vi "Collect file info metadata.vi"(0 "reference in":refnum<class "metadata.lvclass">, 5 "error in (no error)":errorcluster) -> (14 "reference out":refnum<class "metadata.lvclass">, 16 "Metadata":T1, 19 "error out":errorcluster)   [LabVIEW 2019, in "metadata.lvclass"]
uses:
  metadata.lvclass
  Metadata output --cluster.ctl
  Write time and date string --constant.ctl
panel:
  out "Property Names":string[](array[string])
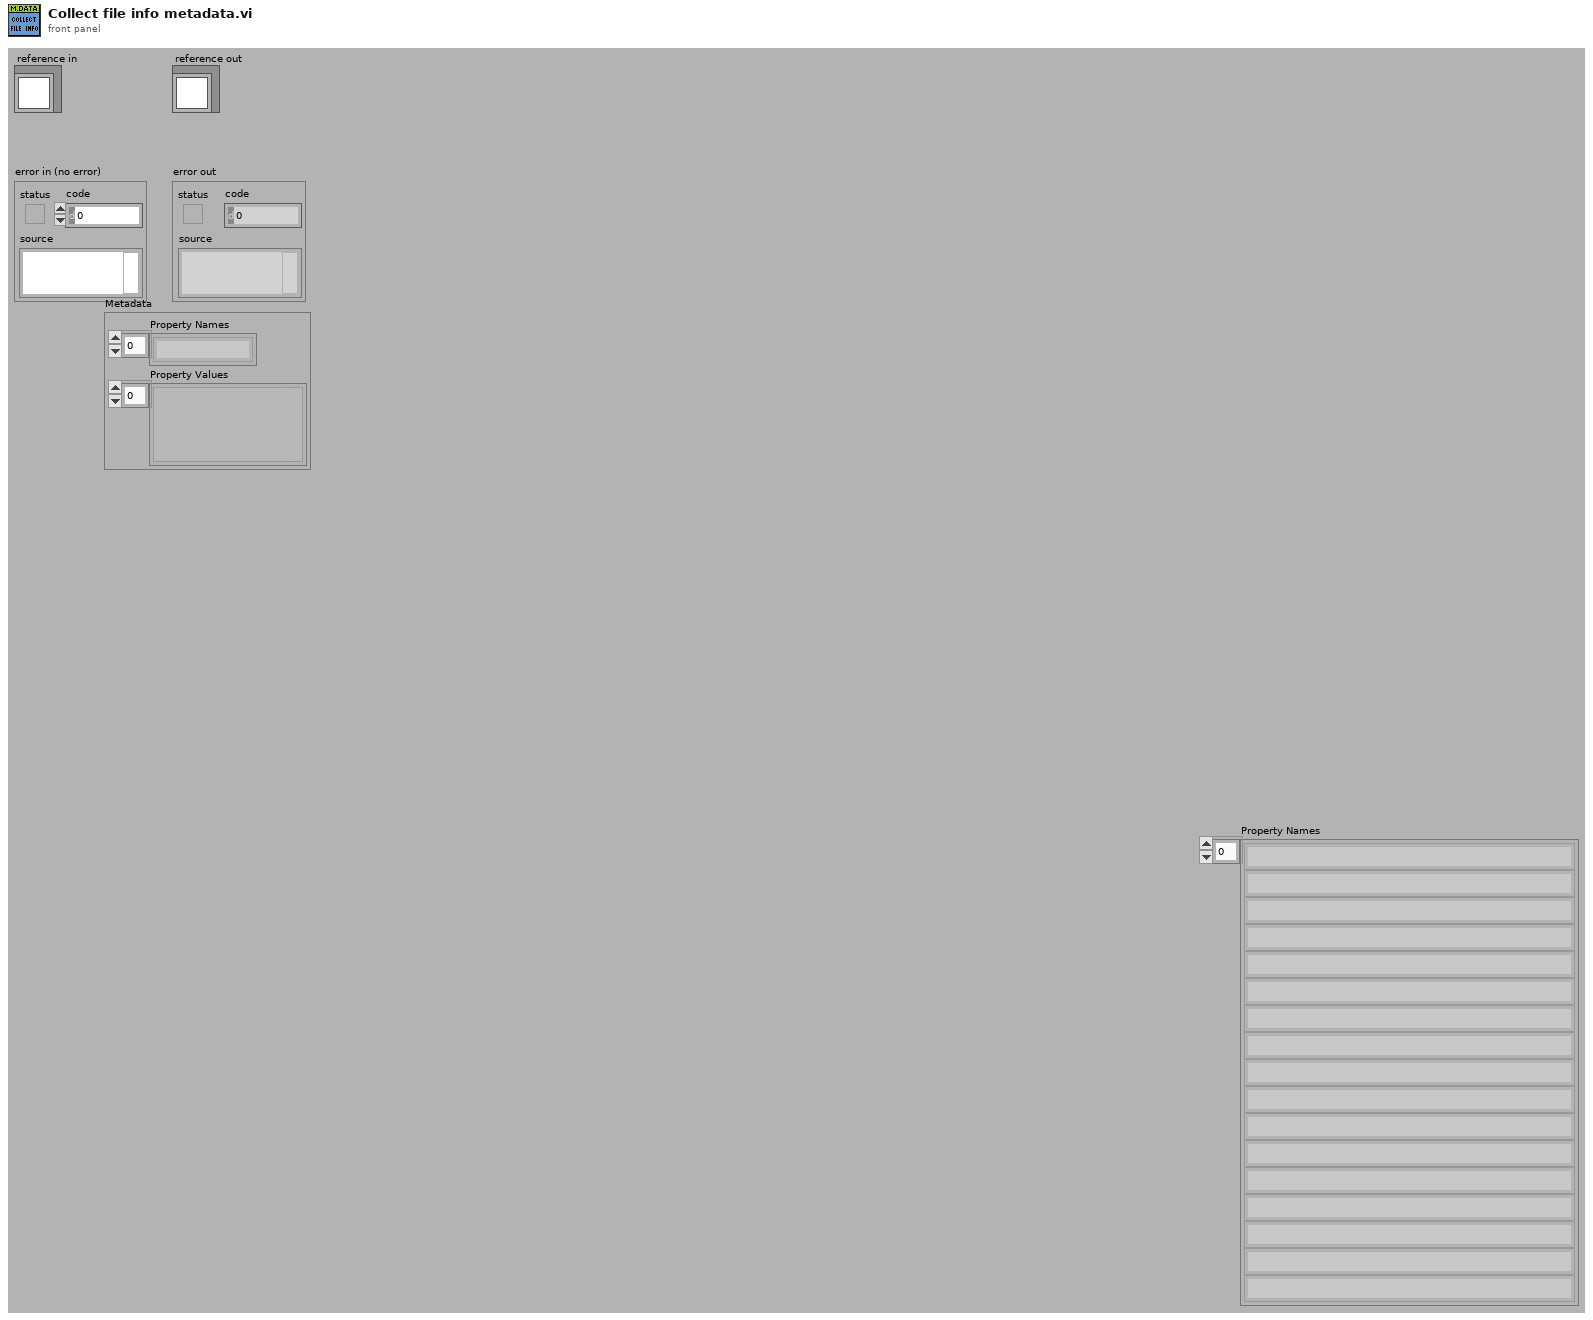
[diagram p1: front panel]
types:
  T1 = typedef "metadata.lvclass/Metadata output --cluster.ctl" = cluster{"Property Names":string[], "Property Values":variant[]}
  T2 = typedef "metadata.lvclass/Write time and date string --constant.ctl" = string
  T3 = typedef "metadata.lvclass/ObjectAttributes.ctl" = cluster{"MyAttribute":dbl, "System Control":T4, "file info":T5, "Sample info":T6, "Cantilever info":T7, "XYZ piezos":T8, "Mapping":T9, "Fcurve segment":T10[], "Fast fpga segment":T12, "Chirp":T13, "precision (6)":i16, "width (-)":i16, "Metadata":T1, "config filepath":path, "Section names []":string[], "Property names []":string[], "nb elements":u16}
  T4 = typedef "metadata.lvclass/System control parameters.ctl" = cluster{"FPGA SW version":string, "TDMS file version":string, "Instrument":string, "Instrument model":string, "Instrument scanner":string, "Instrument clockrate (Mhz)":string, "Instrument tick time (us)":string}
  T5 = typedef "metadata.lvclass/File info parameters.ctl" = cluster{"Time Stamp":timestamp, "Filename":string, "Filepath":path, "User":string, "Experiment_name":string, "Curve_id":string, "number_segments":u8, "number_consecutive_scans":u32}
  T6 = typedef "metadata.lvclass/Sample info parameters.ctl" = cluster{"Sample name":string, "Sample species":string}
  T7 = typedef "metadata.lvclass/Cantilever info parameters.ctl" = cluster{"spring constant calib method":string, "invOLS calib method":string, "thermal calib deflection channel":string, "model":string, "shape":string, "tip geometry":string, "Laser sum (V)":dbl, "Laser power (mA)":dbl, "invOLS_(nm/V)":dbl, "spring constant nominal (N/m)":dbl, "spring constant calib (N/m)":dbl, "resosnance frequency air calib (Hz)":dbl, "resosnance frequency calib (Hz)":dbl, "quality factor":dbl, "Acoefficident_GCI_(nN.s^1.3/m)":dbl, "half angle (deg)":dbl, "tip radius (m)":dbl, "tip height (m)":dbl, "system mount angle (deg)":dbl}
  T8 = typedef "metadata.lvclass/XYZ piezos parameters.ctl" = cluster{"X stage piezo sensitivity (nm/V)":dbl, "X stage piezo gain":dbl, "X velocity (V/tick)":dbl, "X closed loop":bool, "Y stage piezo sensitivity (nm/V)":dbl, "Y stage piezo gain":dbl, "Y velocity (V/tick)":dbl, "Y closed loop":bool, "Z stage piezo sensitivity (nm/V)":dbl, "Z stage piezo gain":dbl, "Z closed loop":bool, "X position (V)":dbl, "Y position (V)":dbl}
  T9 = typedef "metadata.lvclass/Mapping parameters.ctl" = cluster{"Mapping":bool, "index":u16, "position row":u16, "position column":u16, "next position row":i16, "next position column":i16, "X initial position (V)":dbl, "Y initial position (V)":dbl, "X step size (V)":dbl, "Y step size (V)":dbl}
  T10 = typedef "metadata.lvclass/Fcurve segment.ctl" = cluster{"type":T11, "fast_fpga_trigger":bool, "nb":u8, "duration (ticks)":i64, "nb points":i32, "sampling rate (S/s)":u32, "Zpiezo control out":string, "initial deflection (V)":dbl, "relative setpoint":bool, "setpoint on":bool, "setpoint (V)":dbl, "setpoint trigger channel":string, "velocity (V/tick)":dbl, "Z position setpoint trigger (V)":dbl, "Z retract length (V)":dbl, "dec factor":u32}
  T11 = typedef "metadata.lvclass/Segment type--combobox.ctl" = string
  T12 = typedef "metadata.lvclass/fast fpga segment parameters.ctl" = cluster{"Fast start time trigger":timestamp, "nb_points":u32, "sampling_rate_(S/s)":u32, "duration_(ticks)":u32}
  T13 = typedef "metadata.lvclass/Chirp added parameters.ctl" = cluster{"f start (Hz)":dbl, "f end (Hz)":dbl, "Sweep type":string}
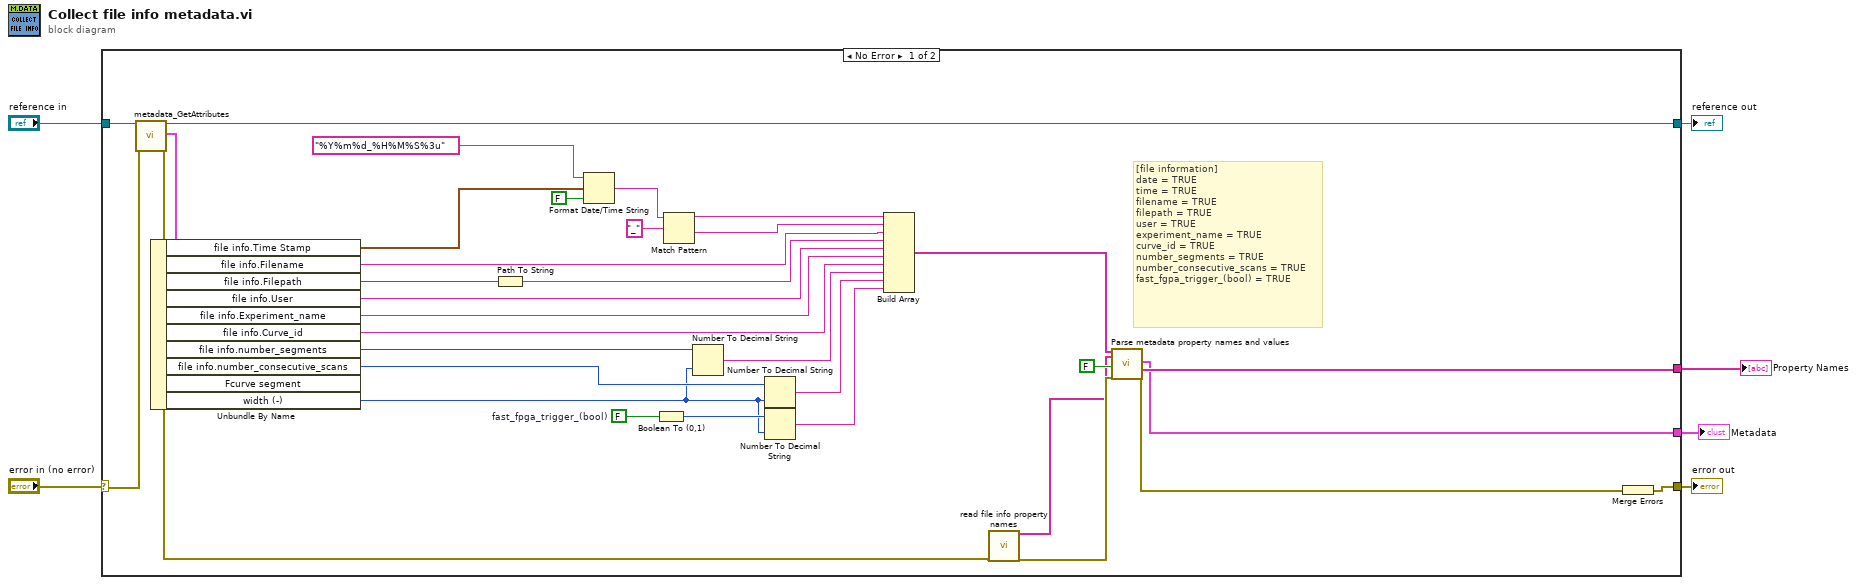
[diagram p0: block diagram]
diagram:
  n1 = case shown="No Error" "error in (no error)" {
    selector: "error in (no error)" -> [w37 w42]
    tunnel: [w40 w42] -> w5
    tunnel: [w38 w41] -> w3
    tunnel: "reference in" -> [w39 w41]
    tunnel: [w34 _] -> w2
    tunnel: [w33 _] -> w1
    frame No Error {
      w7 = FALSE  # fast_fpga_trigger_(bool)
      # "[file information]\ndate = TRUE    \ntime = TRUE    \nfilename = TRUE    \nfilepath = TRUE    \nuser = TRUE  \nexperiment_name = TRUE  \ncurve_id = TRUE\nnumber_segments = TRUE\nnumber_consecutive_scans = TRUE\nfast_fgpa_trigger_(bool) = TRUE"
      n2 = call "metadata_GetAttributes.vi"("reference in"=w39, "error in (no error)"=w37) -> ("reference out"=w38:refnum<class "metadata.lvclass">, "attributes"=w36:T3, "error out"=w14:errorcluster)  [unwired: 14 in, 1 out]
      n3 = Unbundle By Name(w36) -> ("file info.Time Stamp"=w25:timestamp, "file info.Filename"=w23:string, "file info.Filepath"=w21:path, "file info.User"=w20:string, "file info.Experiment_name"=w19:string, "file info.Curve_id"=w18:string, "file info.number_segments"=w17:u8, "file info.number_consecutive_scans"=w16:u32, "width (-)"=w15:i16)  [unwired: 1 out]
      n4 = Path To String(path=w21) -> (string=w22:string)
      n5 = Format Date/Time String(time format string (%c)=T2 "%Y%m%d_%H%M%S%3u", seconds (now)=w25, UTC format=FALSE) -> (date/time string=w31:string)
      n6 = Boolean To (0,1)(Boolean=w7) -> (0, 1=w27:i16)
      n7 = Match Pattern(string=w31, regular expression="_") -> (before substring=w24:string, after substring=w30:string)  [unwired: 1 in, 2 out]
      n8 = Number To Decimal String(number=w17, width (-)=w15) -> (decimal integer string=w29:string)
      n9 = Number To Decimal String(number=w16, width (-)=w15) -> (decimal integer string=w28:string)
      n10 = Number To Decimal String(number=w27, width (-)=w15) -> (decimal integer string=w26:string)
      n11 = Build Array(w24, w30, w23, w22, w20, w19, w18, w29, w28, w26) -> (w10:string[])
      n12 = call "read file info property names.vi"("error in (no error)"=w14) -> ("Property names.File info"=w11:string[], "error out"=w13:errorcluster)  [unwired: 17 in]
      n13 = call "Parse metadata property names and values.vi"("Data intput []"=w10, "property names []"=w11, "List param"=FALSE, "error in (no error)"=w13) -> ("Array"=w34:string[], "output cluster"=w33:T1, "error out"=w35:errorcluster)  [unwired: 12 in, 1 out]
      n14 = Merge Errors(w35) -> (w40:errorcluster)
    }
    frame Error {
    }
  }
  "error out" <- w5
  "reference out" <- w3
  "Property Names" <- w2
  "Metadata" <- w1
